vi "Trav_pos_for_Email.vi"() -> (0 "String":string)   [LabVIEW 2021]
uses:
  Controls/Overhead.ctl
  Globals/Trav_pos_global.vi
  Route mapping/Route_mapping_global.vi
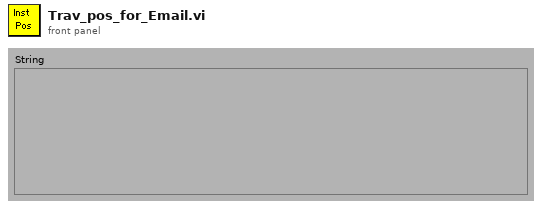
[diagram p1: front panel]
types:
  T1 = typedef "Overhead.ctl" = enum16{"Update total times", "Read Current Overhead", "Re Scale totals to 3 hrs", "Initialise totals to 3hr"}
  T2 = typedef "Tunnel_Coordinates.ctl" = enum16{"Work in Tunnel Coordinates", "Work in Model Coordinates"}
  T3 = typedef "Traverse_cluster.ctl" = cluster{"Start X":sgl, "Start Y":sgl, "Start Z":sgl, "End X":sgl, "End Y":sgl, "End Z":sgl, "nPoints":i32, "Spacing":T4, "Filename":path, "Tunnel Speed":dbl, "Averaging time (mins)":dbl, "Extra Commands":string, "Carrier_1 Q (l/min)":dbl, "Carrier_2 Q (l/min)":dbl, "Trace Gas Concentration (%)":dbl, "Specific Arguments":string, "Comments":string, "Row No":i32, "Row Type Selector":T5, "EstCompl":string, "Row Duration (mins)":dbl, "nValidPoints":i32, "Meas Setup File":string}
  T4 = typedef "Spacing.ctl" = enum16{"Linear", "Log", "Gauss", "Specified", "N/A"}
  T5 = typedef "Multi_run_mode.ctl" = enum16{"Move Traverse Only", "Set Tunnel Speed Only", "Set Source Only", "Set Measurement Conditions", "Single Measurement", "Vertical Profile", "Lateral Profile", "Longitudinal Profile", "Multi-Axis Profile", "Explore Volume", "Auto Calibrate", "Meas Fast FID Bkgnd", "Check Beam Power", "Scanning Valve Measurement", "Run VI Named:", "Set ADAM Ch", "Wait (minutes)", "Send Message", "Synchronize With:", "Fall Back to this Row", "Turn Off Row Repeating", "Traverse 3D Volume", "Blank Row", "Jump to Fall Back Row"}
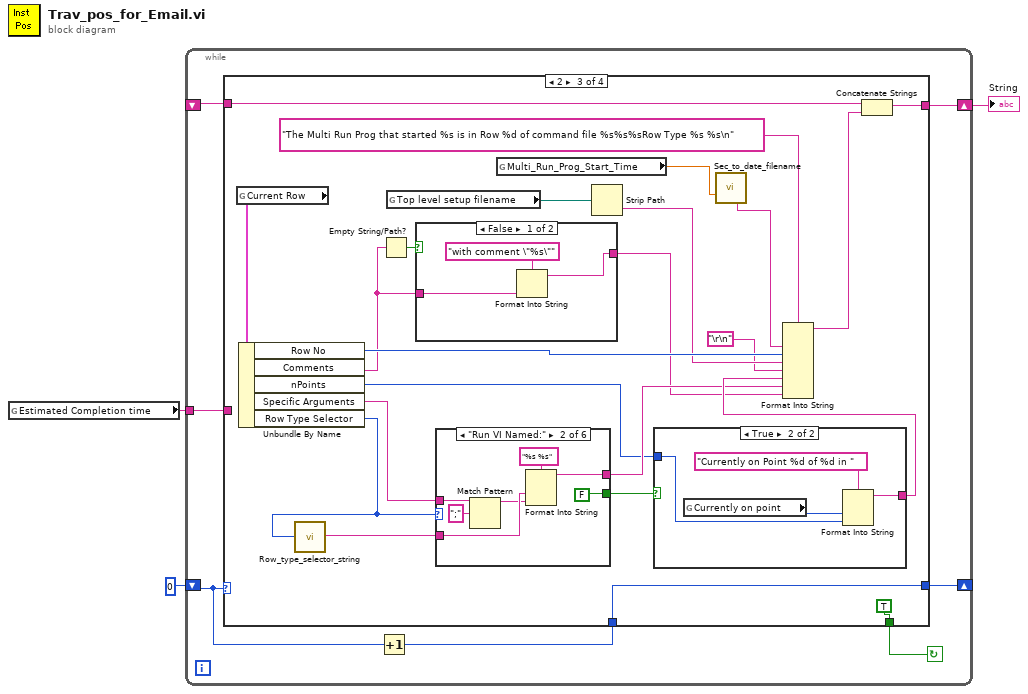
[diagram p0: block diagram]
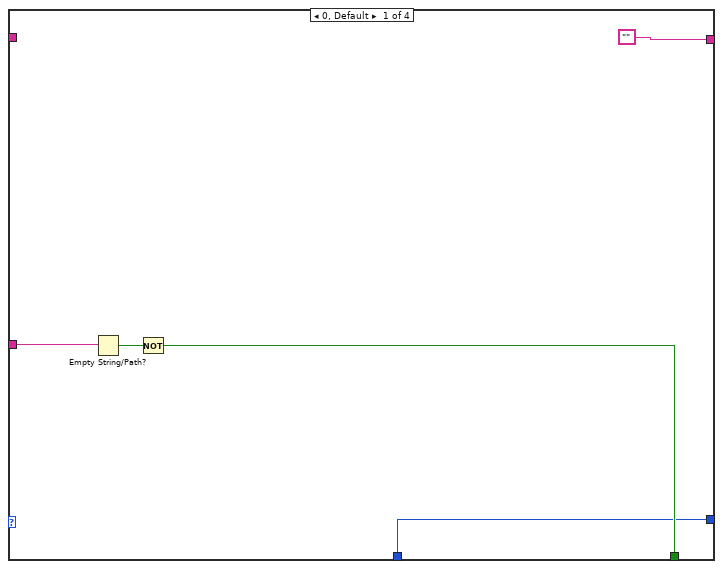
[diagram p2: hidden frame]
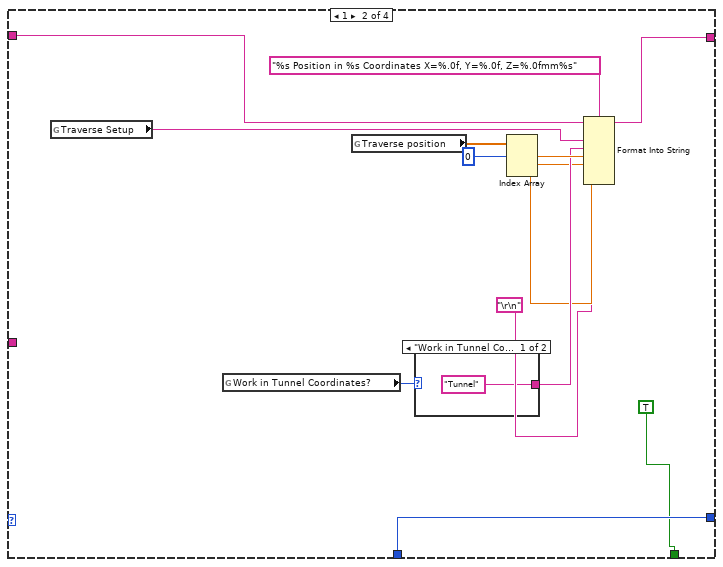
[diagram p3: hidden frame]
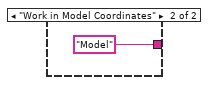
[diagram p4: hidden frame]
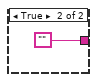
[diagram p5: hidden frame]
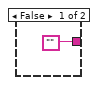
[diagram p6: hidden frame]
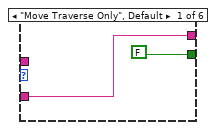
[diagram p7: hidden frame]
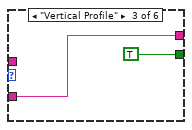
[diagram p8: hidden frame]
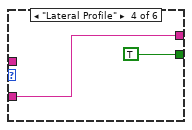
[diagram p9: hidden frame]
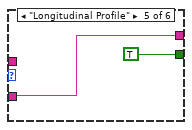
[diagram p10: hidden frame]
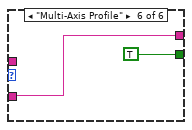
[diagram p11: hidden frame]
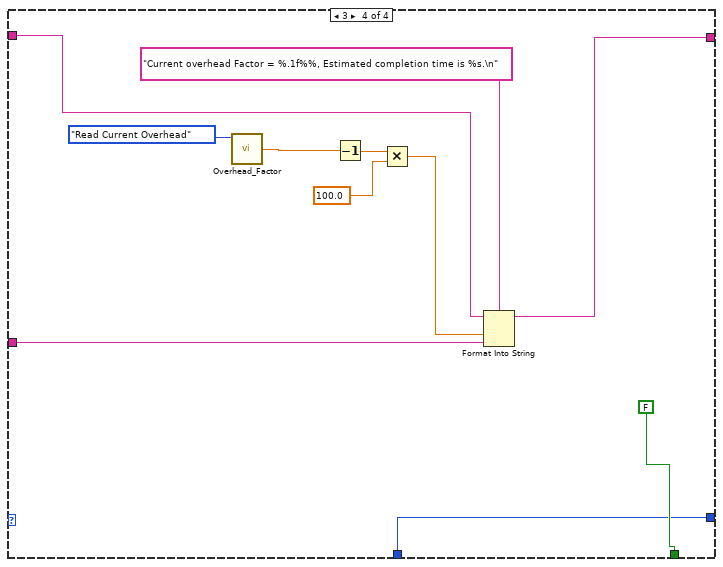
[diagram p12: hidden frame]
diagram:
  n1 = global read "Trav_pos_global.vi" "Estimated Completion time"() -> (w1:string)
  n2 = while {
    shift-left: _ -> [w5]
    shift-right: [w7] -> w2
    shift-left: 0 -> [w10]
    shift-right: [w9] -> _
    tunnel: w1 -> [w4]
    stop <- w6 continue-if-true
    n3 = Increment(x=w10) -> (x+1=w8:i32)
    n4 = case shown="2" w10 {
      tunnel: [w12 w29 w49 w90] -> w9
      tunnel: w8 -> [w12 w29 w49 w90]
      tunnel: ["" w24 w54 w82] -> w7
      tunnel: [w13 TRUE TRUE FALSE] -> w6
      tunnel: w5 -> [_ w25 w37 w83]
      tunnel: w4 -> [w15 _ _ w81]
      frame 0, Default {
        n5 = Empty String/Path?(string/path=w15) -> (empty?=w14:bool)
        n6 = Not(x=w14) -> (.not. x?=w13:bool)
      }
      frame 1 {
        n7 = global read "Route_mapping_global.vi" "Traverse Setup"() -> (w17:string)
        n8 = global read "Trav_pos_global.vi" "Work in Tunnel Coordinates?"() -> (w23:T2)
        n9 = global read "Trav_pos_global.vi" "Traverse position"() -> (w20:sgl[])
        n10 = case shown="\"Work in Tunnel Coordinates\"" w23 {
          tunnel: ["Tunnel" "Model"] -> w21
          frame "Work in Tunnel Coordinates" {
          }
          frame "Work in Model Coordinates" {
          }
        }
        n11 = Index Array(array=w20, index #1=0 ("index")) -> (element #1=w22:sgl, element #2=w19:sgl, element #3=w18:sgl)  [unwired: 2 in]
        n12 = Format Into String(format string="%s Position in %s Coordinates X=%.0f, Y=%.0f, Z=%.0fmm%s" ("Format String"), initial string=w25, w17, w21, w22, w19, w18, "\r\n") -> (resulting string=w24:string)  [unwired: 1 in, 1 out]
      }
      frame 2 {
        n13 = global read "Trav_pos_global.vi" "Current Row"() -> (w46:T3)
        n14 = Unbundle By Name(w46) -> ("Row No"=w53:i32, "Comments"=w34:string, "nPoints"=w41:i32, "Specific Arguments"=w43:string, "Row Type Selector"=w42:T5)
        n15 = call "Row_type_selector_string.vi"("Mode"=w42) -> ("Output string"=w45:string)
        n16 = Empty String/Path?(string/path=w34) -> (empty?=w36:bool)
        n17 = global read "Trav_pos_global.vi" "Top level setup filename"() -> (w40:path)
        n18 = case shown="False" w36 {
          tunnel: [w55 ""] -> w35
          tunnel: w34 -> [w57 _]
          frame False {
            n19 = Format Into String(format string="with comment \"%s\"", w57) -> (resulting string=w55:string)  [unwired: 2 in, 1 out]
          }
          frame True {
          }
        }
        n20 = case shown="\"Run VI Named:\"" w42 {
          tunnel: [FALSE FALSE TRUE TRUE TRUE TRUE] -> w52
          tunnel: w45 -> [w64 w71 w73 w75 w77 w79]
          tunnel: [w64 w69 w73 w75 w77 w79] -> w44
          tunnel: w43 -> [_ w67 _ _ _ _]
          frame "Move Traverse Only", Default {
          }
          frame "Run VI Named:" {
            n21 = Match Pattern(string=w67, regular expression=";") -> (before substring=w66:string)  [unwired: 4 out]
            n22 = Format Into String(format string="%s %s" ("Format String"), w71, w66) -> (resulting string=w69:string)  [unwired: 2 in, 1 out]
          }
          frame "Vertical Profile" {
          }
          frame "Lateral Profile" {
          }
          frame "Longitudinal Profile" {
          }
          frame "Multi-Axis Profile" {
          }
        }
        n23 = global read "Trav_pos_global.vi" "Multi_Run_Prog_Start_Time"() -> (w33:dbl)
        n24 = Strip Path(path=w40) -> (name=w39:string)  [unwired: 1 out]
        n25 = case shown="True" w52 {
          tunnel: w41 -> [_ w62]
          tunnel: ["" w60] -> w48
          frame False {
          }
          frame True {
            n26 = global read "Trav_pos_global.vi" "Currently on point"() -> (w63:i32)
            n27 = Format Into String(format string="Currently on Point %d of %d in " ("Format String"), w63, w62) -> (resulting string=w60:string)  [unwired: 2 in, 1 out]
          }
        }
        n28 = call "Sec_to_date_filename.vi"("ss1904"=w33) -> ("YYYY-mm-DD HH:MM"=w32:string)  [unwired: 5 in, 9 out]
        n29 = Format Into String(format string="The Multi Run Prog that started %s is in Row %d of command file %s%s%sRow Type %s %s\n" ("Format String"), w32, w53, w39, "\r\n", w48, w44, w35) -> (resulting string=w47:string)  [unwired: 2 in, 1 out]
        n30 = Concatenate Strings(w37, w47) -> (w54:string)
      }
      frame 3 {
        n31 = call "Overhead_Factor.vi"("Mode"=Overhead."Read Current Overhead") -> ("Current Overhead Factor"=w88:dbl)  [unwired: 3 in]
        n32 = Decrement(x=w88) -> (x-1=w87:dbl)
        n33 = Multiply(x=w87, y=100.0) -> (x*y=w85:dbl)
        n34 = Format Into String(format string="Current overhead Factor = %.1f%%, Estimated completion time is %s.\n" ("Format String"), initial string=w83, w85, w81) -> (resulting string=w82:string)  [unwired: 1 in, 1 out]
      }
    }
  }
  "String" <- w2
